vi "FibrePhotometry_Ephys_ver2_SubVersion.vi"(4 "RecDur (min)":dbl, 6 "Raw samples per s":dbl=2000.0 min=1000.0 max=2000.0, 7 "Dir":string="C:\\Test", 8 "Frequency":dbl=40.0, 9 "Duty cycle (%)":dbl=50.0, 10 "470 LED power":dbl=2.0 min=0.0 max=5.0, 11 "405 LED Power":dbl=1.0 min=0.0 max=5.0) -> ()   [LabVIEW 2017]
uses:
  <vilib>/DAQmx/read.llb/DAQmx Read (Analog 2D DBL NChan NSamp).vi
  <vilib>/DAQmx/write.llb/DAQmx Write (Analog 1D DBL NChan 1Samp).vi
  <vilib>/DAQmx/miscellaneous.llb/DAQmx Fill In Error Info.vi
  <vilib>/DAQmx/create/channels.llb/DAQmx Create Channel (AO-Voltage-Basic).vi
panel:
  out "Raw":dbl[][](graph)
  in  "Amplification Factor":dbl=1.0 format="%#_13g"
  out "Start Time":u32
  out "Recording Time (sec)":dbl
  out "Save Path":path
  out "Processed Data":dbl[][](graph)
  out "SyncPulses":waveform(dbl)[](graph)
  in  "Emergency Stop":bool
  out "Loop Time":u32
  in  "Comments":string
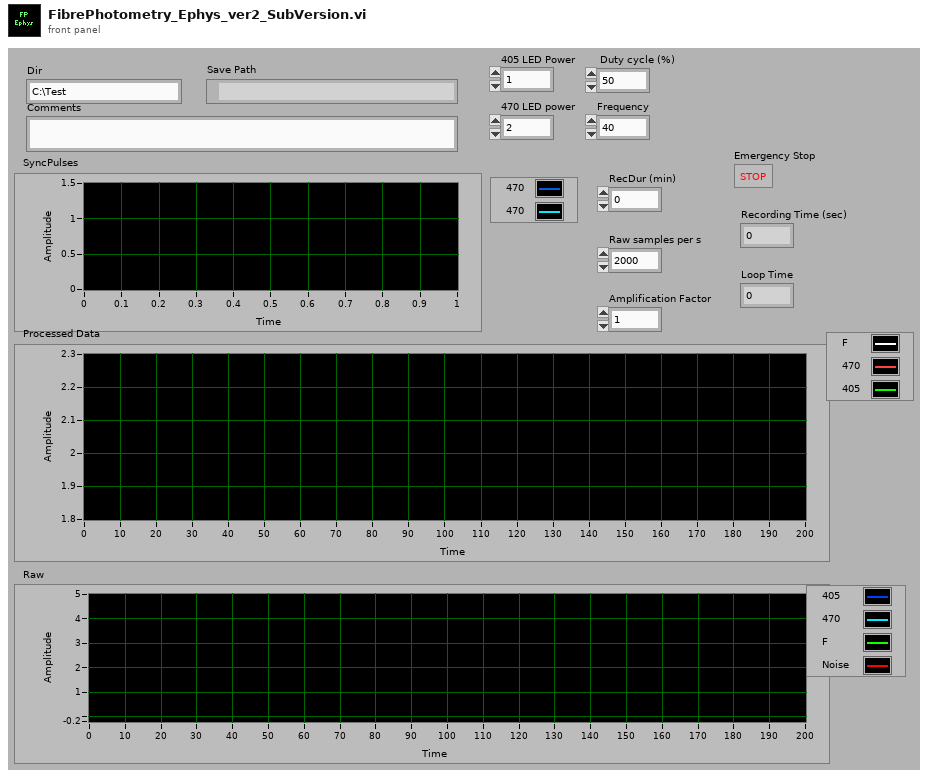
[diagram p1: front panel]
types:
  T1 = enum16{"big-endian, network order", "native, host order", "little-endian"}
  T2 = cluster{"Comments":string, "Dir":string, "Frequency":dbl, "470 LED power":dbl, "405 LED Power":dbl, "Raw samples per s":dbl, " Duty cycle (%)":dbl}
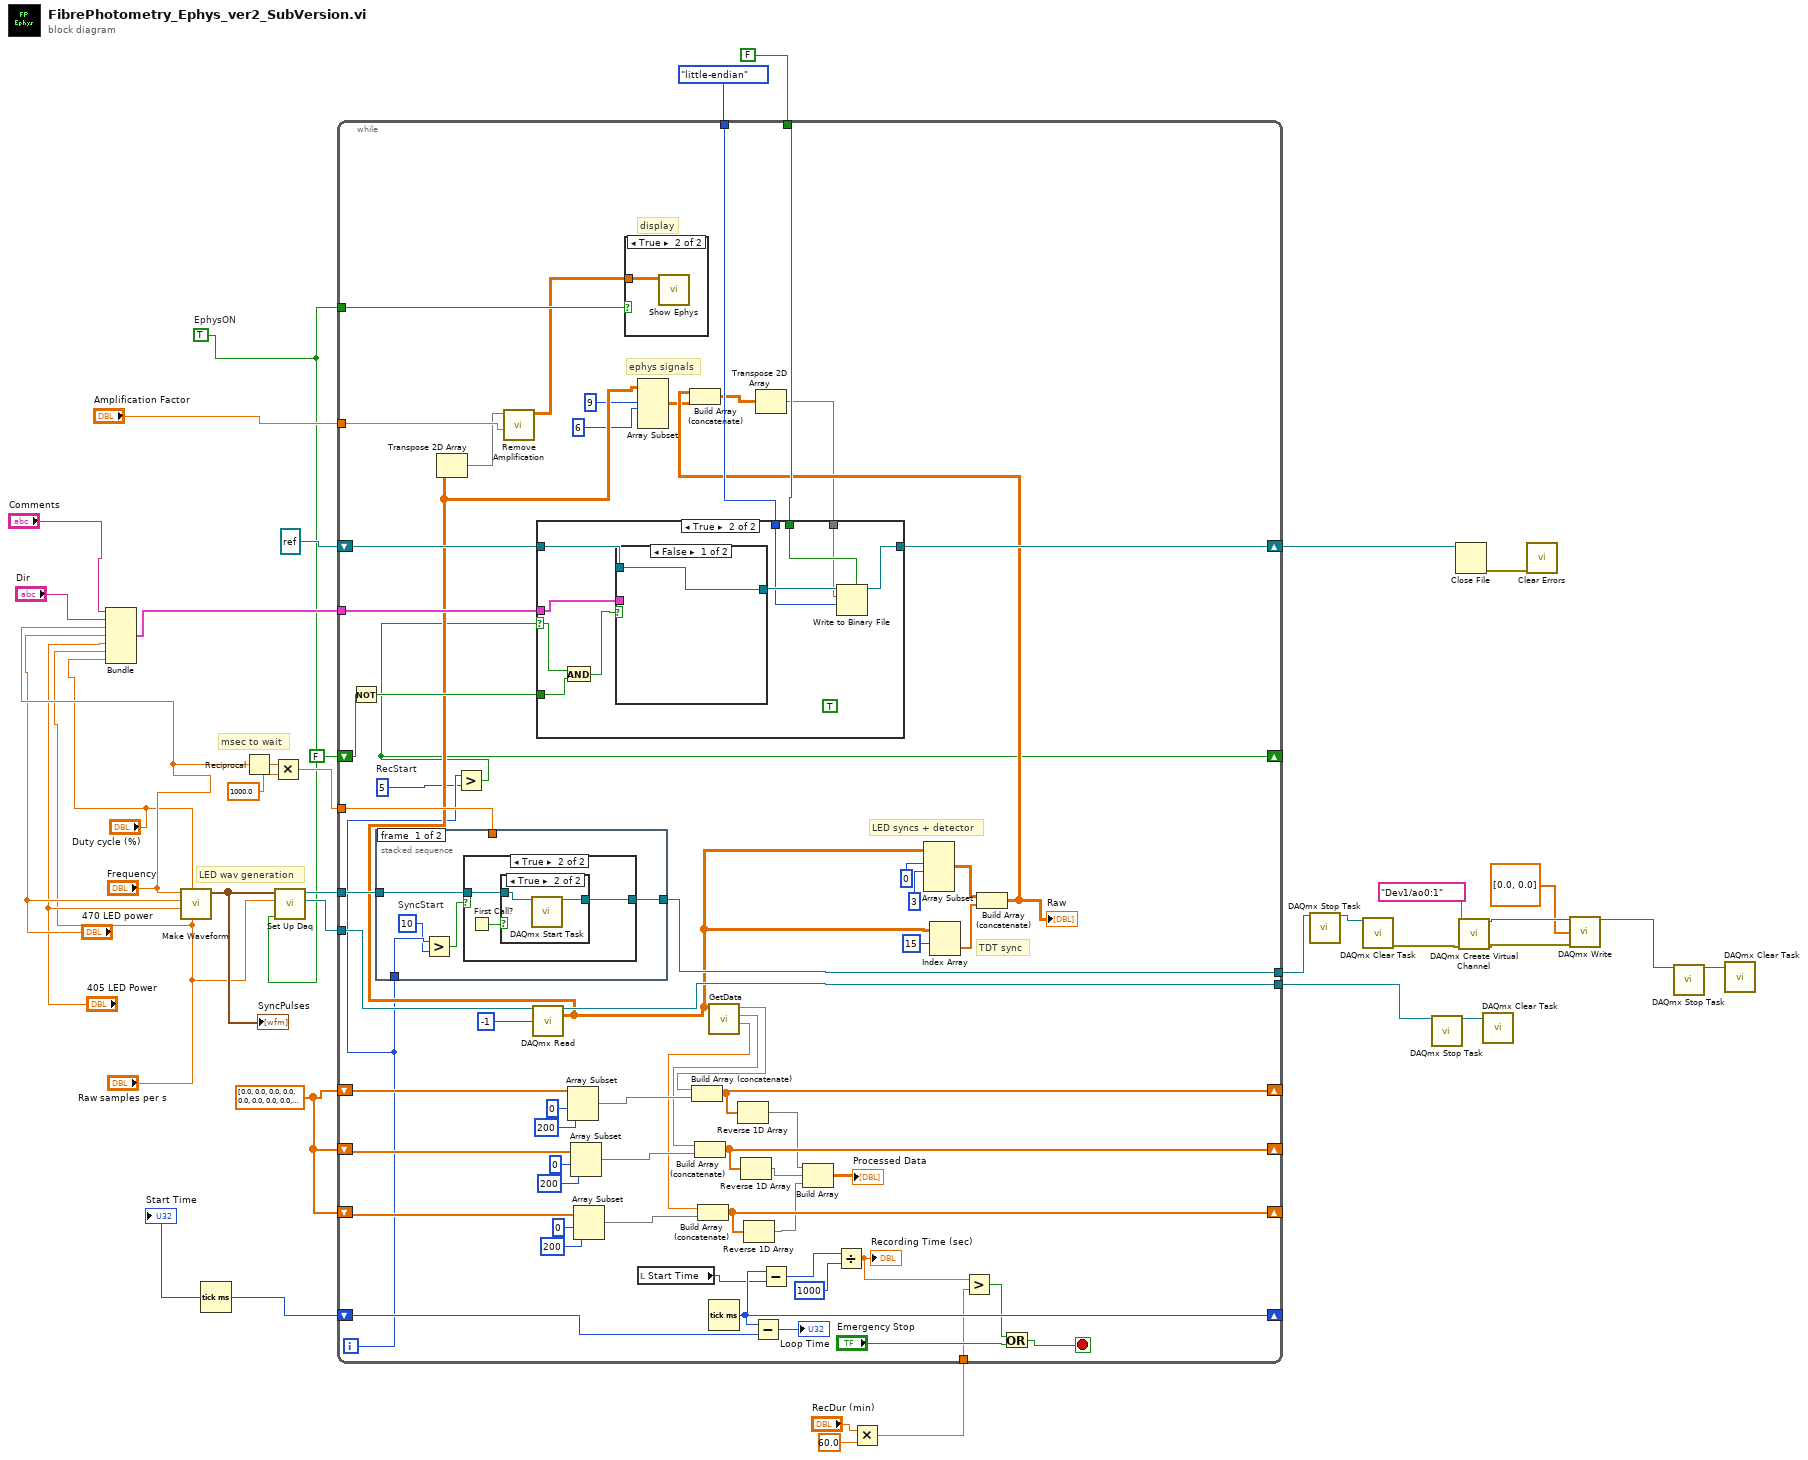
[diagram p0: block diagram]
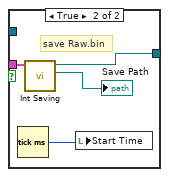
[diagram p4: hidden frame]
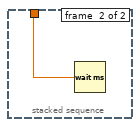
[diagram p7: hidden frame]
diagram:
  w4 = TRUE  # EphysON
  w13 = dbl[] [0.0, 0.0, 0.0, 0.0, 0.0, 0.0, 0.0, 0.0, 0.0, 0.0, 0.0, 0.0, 0.0, 0.0, 0.0, 0.0, 0.0, 0.0, 0.0, 0.0, 0.0, 0.0, 0.0, 0.0, 0.0, 0.0, 0.0, 0.0, 0.0, 0.0, 0.0, 0.0, 0.0, 0.0, 0.0, 0.0, 0.0, 0.0, 0.0, 0.0, 0.0, 0.0, 0.0, 0.0, 0.0, 0.0, 0.0, 0.0, 0.0, 0.0, 0.0, 0.0, 0.0, 0.0, 0.0, 0.0, 0.0, 0.0, 0.0, 0.0, 0.0, 0.0, 0.0, 0.0, 0.0, 0.0, 0.0, 0.0, 0.0, 0.0, 0.0, 0.0, 0.0, 0.0, 0.0, 0.0, 0.0, 0.0, 0.0, 0.0, 0.0, 0.0, 0.0, 0.0, 0.0, 0.0, 0.0, 0.0, 0.0, 0.0, 0.0, 0.0, 0.0, 0.0, 0.0, 0.0, 0.0, 0.0, 0.0, 0.0, 0.0, 0.0, 0.0, 0.0, 0.0, 0.0, 0.0, 0.0, 0.0, 0.0, 0.0, 0.0, 0.0, 0.0, 0.0, 0.0, 0.0, 0.0, 0.0, 0.0, 0.0, 0.0, 0.0, 0.0, 0.0, 0.0, 0.0, 0.0, 0.0, 0.0, 0.0, 0.0, 0.0, 0.0, 0.0, 0.0, 0.0, 0.0, 0.0, 0.0, 0.0, 0.0, 0.0, 0.0, 0.0, 0.0, 0.0, 0.0, 0.0, 0.0, 0.0, 0.0, 0.0, 0.0, 0.0, 0.0, 0.0, 0.0, 0.0, 0.0, 0.0, 0.0, 0.0, 0.0, 0.0, 0.0, 0.0, 0.0, 0.0, 0.0, 0.0, 0.0, 0.0, 0.0, 0.0, 0.0, 0.0, 0.0, 0.0, 0.0, 0.0, 0.0, 0.0, 0.0, 0.0, 0.0, 0.0, 0.0, 0.0, 0.0, 0.0, 0.0, 0.0, 0.0, 0.0, 0.0, 0.0, 0.0, 0.0, 0.0, 0.0]
  # "msec to wait"
  # "LED wav generation"
  n1 = Bundle("Comments"="Comments", "Dir"="Dir", "Frequency"="Frequency", "470 LED power"="470 LED power", "405 LED Power"="405 LED Power", "Raw samples per s"="Raw samples per s", "Duty cycle (%)"="Duty cycle (%)") -> (w20:T2)  [unwired: 1 in]
  n2 = call "Make Waveform.vi"("Number of samples per s"="Raw samples per s", "Duty cycle (%)"="Duty cycle (%)", "405 LED Power"="405 LED Power", "470 LED power"="470 LED power", "Frequency"="Frequency") -> ("Array"=w30:waveform(dbl)[])  [unwired: 6 in]
  "SyncPulses" <- w30
  n3 = Tick Count (ms)() -> (millisecond timer value=w32:u32)
  "Start Time" <- w32
  n4 = Reciprocal(x="Frequency") -> (1/x=w36:dbl)
  n5 = Multiply(x=w36, y=1000.0) -> (x*y=w34:dbl)
  n6 = call "Set Up Daq.vi"("Use Ephys"=w4, "Number of samples per s"="Raw samples per s", "Array"=w30) -> ("task out 2"=w37:refnum<k21>, "Refnum out"=w38:refnum<k21>)  [unwired: 7 in]
  n7 = Multiply(x="RecDur (min)", y=60.0) -> (x*y=w1:dbl)
  n8 = while {
    tunnel: w38 -> [w103]
    tunnel: w37 -> [w101]
    tunnel: w34 -> [w102]
    shift-right: [w70] -> w17
    shift-left: refnum<file> refnum ("refnum out") -> [w71]
    tunnel: [w99] -> w31
    shift-right: [w95] -> _
    shift-left: w13 -> [w94]
    shift-right: [w87] -> _
    shift-left: w13 -> [w84]
    shift-right: [w86] -> _
    shift-left: w13 -> [w85]
    shift-right: [w79] -> _
    shift-left: w32 -> [w80]
    tunnel: FALSE ("prepend array or string size? (T)") -> [w69]
    tunnel: T1."little-endian" ("byte order (0:big-endian, network order)") -> [w68]
    tunnel: w20 -> [w67]
    shift-right: [w44] -> _
    shift-left: FALSE ("Recording") -> [w65]
    tunnel: w4 -> [w63]
    tunnel: "Amplification Factor" -> [w61]
    tunnel: [w58] -> w5
    tunnel: w1 -> [w40]
    i -> [w46]
    stop <- w42 stop-if-true
    w45 = 5  # RecStart
    # "ephys signals"
    # "LED syncs + detector"
    # "TDT sync"
    # "display"
    n9 = Not(x=w65) -> (.not. x?=w64:bool)
    n10 = stacked-sequence {
      tunnel: w103 -> [w125 _]
      tunnel: [w124 _] -> w58
      tunnel: w102 -> [_ w133]
      tunnel: w46 -> [w123 _]
      frame #0 {
        w122 = 10  # SyncStart
        n11 = Greater?(x=w123, y=w122) -> (0:w121:bool)
        n12 = case shown="True" w121 {
          tunnel: w125 -> [w126 w128]
          tunnel: [w126 w127] -> w124
          frame False {
          }
          frame True {
            n13 = First Call?() -> (First Call?: T/F=w129:bool)
            n14 = case shown="True" w129 {
              tunnel: w128 -> [w130 w132]
              tunnel: [w130 w131] -> w127
              frame False {
              }
              frame True {
                n15 = call <vilib>:"DAQmx Start Task.vi"("task/channels in"=w132) -> ("task out"=w131:refnum<k21>)  [unwired: 13 in, 1 out]
              }
            }
          }
        }
      }
      frame #1 {
        n16 = Wait (ms)(milliseconds to wait=w133) -> ()  [unwired: 1 out]
      }
    }
    n17 = Greater?(x=w46, y=w45) -> (0:w44:bool)
    n18 = call-poly <vilib>:"DAQmx Read.vi"("task/channels in"=w101, "number of samples per channel"=-1) -> ("task out"=w99:refnum<k21>, "data"=w53:dbl[][])  [unwired: 11 in, 1 out]
    n19 = Transpose 2D Array(2D array=w53) -> (transposed array=w57:dbl[][])
    n20 = call "Remove Amplification.vi"("Amplification Factor"=w61, "Array"=w57) -> ("Array 2"=w62:dbl[][])  [unwired: 9 in]
    n21 = Array Subset(array=w94, index=0, length=200) -> (w96:dbl[])
    n22 = Array Subset(array=w84, index=0, length=200) -> (w91:dbl[])
    n23 = Array Subset(array=w85, index=0, length=200) -> (w88:dbl[])
    n24 = case shown="True" w63 {
      tunnel: w62 -> [_ w104]
      frame False {
      }
      frame True {
        n25 = call "Show Ephys.vi"("Array"=w104) -> ()  [unwired: 11 in]
      }
    }
    n26 = Array Subset(array=w53, index (row)=9 ("disabled index (col)"), length (row)=6 ("length")) -> (w49:dbl[][])  [unwired: 2 in]
    n27 = local read "Start Time"() -> (w66:u32)
    n28 = call "GetData.vi"("data"=w53) -> ("mean 405"=w75:dbl, "mean 470"=w76:dbl, "F470-F405/F405"=w77:dbl)  [unwired: 8 in]
    n29 = Build Array (concatenate)(w77, w96) -> (w95:dbl[])
    n30 = Build Array (concatenate)(w76, w91) -> (w87:dbl[])
    n31 = Build Array (concatenate)(w75, w88) -> (w86:dbl[])
    n32 = Tick Count (ms)() -> (millisecond timer value=w79:u32)
    n33 = Reverse 1D Array(array=w95) -> (reversed array=w82:dbl[])
    n34 = Reverse 1D Array(array=w87) -> (reversed array=w83:dbl[])
    n35 = Reverse 1D Array(array=w86) -> (reversed array=w81:dbl[])
    n36 = Subtract(x=w79, y=w80) -> (x-y=→"Loop Time":u32)
    n37 = Subtract(x=w79, y=w66) -> (x-y=w73:u32)
    n38 = Build Array(w82, w83, w81) -> (→"Processed Data":dbl[][])
    n39 = Divide(x=w73, y=u32 1000) -> (x/y=w41:dbl)
    "Recording Time (sec)" <- w41
    n40 = Array Subset(array=w53, index (row)=0, length (row)=3 ("length")) -> (w55:dbl[][])  [unwired: 2 in]
    n41 = Index Array(array=w53, index (row)=15) -> (element=w54:dbl[])  [unwired: 1 in]
    n42 = Greater?(x=w41, y=w40) -> (0:w39:bool)
    n43 = Build Array (concatenate)(w55, w54) -> (w50:dbl[][])
    "Raw" <- w50
    n44 = Build Array (concatenate)(w50, w49) -> (w48:dbl[][])
    n45 = Transpose 2D Array(2D array=w48) -> (transposed array=w47:dbl[][])
    n46 = case shown="True" w44 {
      selector: w44 -> [_ w108]
      tunnel: w71 -> [w105 w115]
      tunnel: [w105 w113] -> w70
      tunnel: w69 -> [_ w112]
      tunnel: w68 -> [_ w111]
      tunnel: w67 -> [_ w110]
      tunnel: w64 -> [_ w109]
      tunnel: w47 -> [_ w106]
      frame False {
      }
      frame True {
        (unwired) TRUE ("append to file? (new file:F)")
        n47 = And(x=w108, y=w109) -> (x .and. y?=w107:bool)
        n48 = case shown="False" w107 {
          tunnel: w115 -> [w116 _]
          tunnel: [w116 w120] -> w114
          tunnel: w110 -> [_ w119]
          frame False {
          }
          frame True {
            # "save Raw.bin"
            n49 = Tick Count (ms)() -> (millisecond timer value=w117:u32)
            n50 = call "Int Saving.vi"("Cluster"=w119) -> ("created path"=→"Save Path":path, "Byte Stream File out"=w120:refnum<file>)  [unwired: 8 in, 1 out]
            n51 = local write "Start Time"(w117) -> ()
          }
        }
        n52 = Write to Binary File(file (use dialog)=w114, data=w106, 5:w112, 9:w111) -> (refnum out=w113:refnum<file>)  [unwired: 2 in, 2 out]
      }
    }
    n53 = Or(x=w39, y="Emergency Stop") -> (x .or. y?=w42:bool)
  }
  n54 = call <vilib>:"DAQmx Stop Task.vi"("task/channels in"=w5) -> ("task out"=w12:refnum<k21>)  [unwired: 13 in, 1 out]
  n55 = call <vilib>:"DAQmx Clear Task.vi"("task in"=w12) -> ("error out"=w11:errorcluster)  [unwired: 14 in]
  n56 = call <vilib>:"DAQmx Stop Task.vi"("task/channels in"=w31) -> ("task out"=w33:refnum<k21>)  [unwired: 13 in, 1 out]
  n57 = Close File(refnum=w17) -> (error out=w16:errorcluster)  [unwired: 1 in, 1 out]
  n58 = call-poly <vilib>:"DAQmx Create Virtual Channel.vi"("physical channels"=tag "Dev1/ao0:1", "error in"=w11) -> ("task out"=w8:refnum<k21>, "error out"=w9:errorcluster)  [unwired: 12 in]
  n59 = call <vilib>:"DAQmx Clear Task.vi"("task in"=w33) -> ()  [unwired: 14 in, 1 out]
  n60 = call <vilib>:"Clear Errors.vi"("error in (no error)"=w16) -> ()  [unwired: 5 in, 2 out]
  n61 = call-poly <vilib>:"DAQmx Write.vi"("task/channels in"=w8, "data"=dbl[] [0.0, 0.0], "error in"=w9) -> ("task out"=w6:refnum<k21>)  [unwired: 10 in, 2 out]
  n62 = call <vilib>:"DAQmx Stop Task.vi"("task/channels in"=w6) -> ("task out"=w29:refnum<k21>)  [unwired: 13 in, 1 out]
  n63 = call <vilib>:"DAQmx Clear Task.vi"("task in"=w29) -> ()  [unwired: 14 in, 1 out]
